vi "BinaryAnalysis.vi"() -> ()   [LabVIEW 2018]
uses:
  <vilib>/Utility/file.llb/Write Delimited Spreadsheet (DBL).vi
panel:
  in  "Save Data?":bool
  in  "Directory to Save Data":path=path "C:/Users/Cletus/Desktop/VMI Scan/100218"
  in  "File Name":path=path "test.txt"
  in  "Step Size":dbl format="%#_13g"
  in  "Initial WL":dbl format="%#_13g"
  in  "length":i32=1000
  in  "index":i32
  in  "Custom Marker Colors":u32[](array[colorbox])=[16714752, 16748562, 16773418]
  in  "Update Marker Colors":bool
  out "Intensity Graph":dbl[][](graph)
  in  "Number of Points/Scan":i32
  out "Waveform Graph":waveform(dbl)(graph)
  out "error out":errorcluster
  in  "Binary File Location (.dat)":path
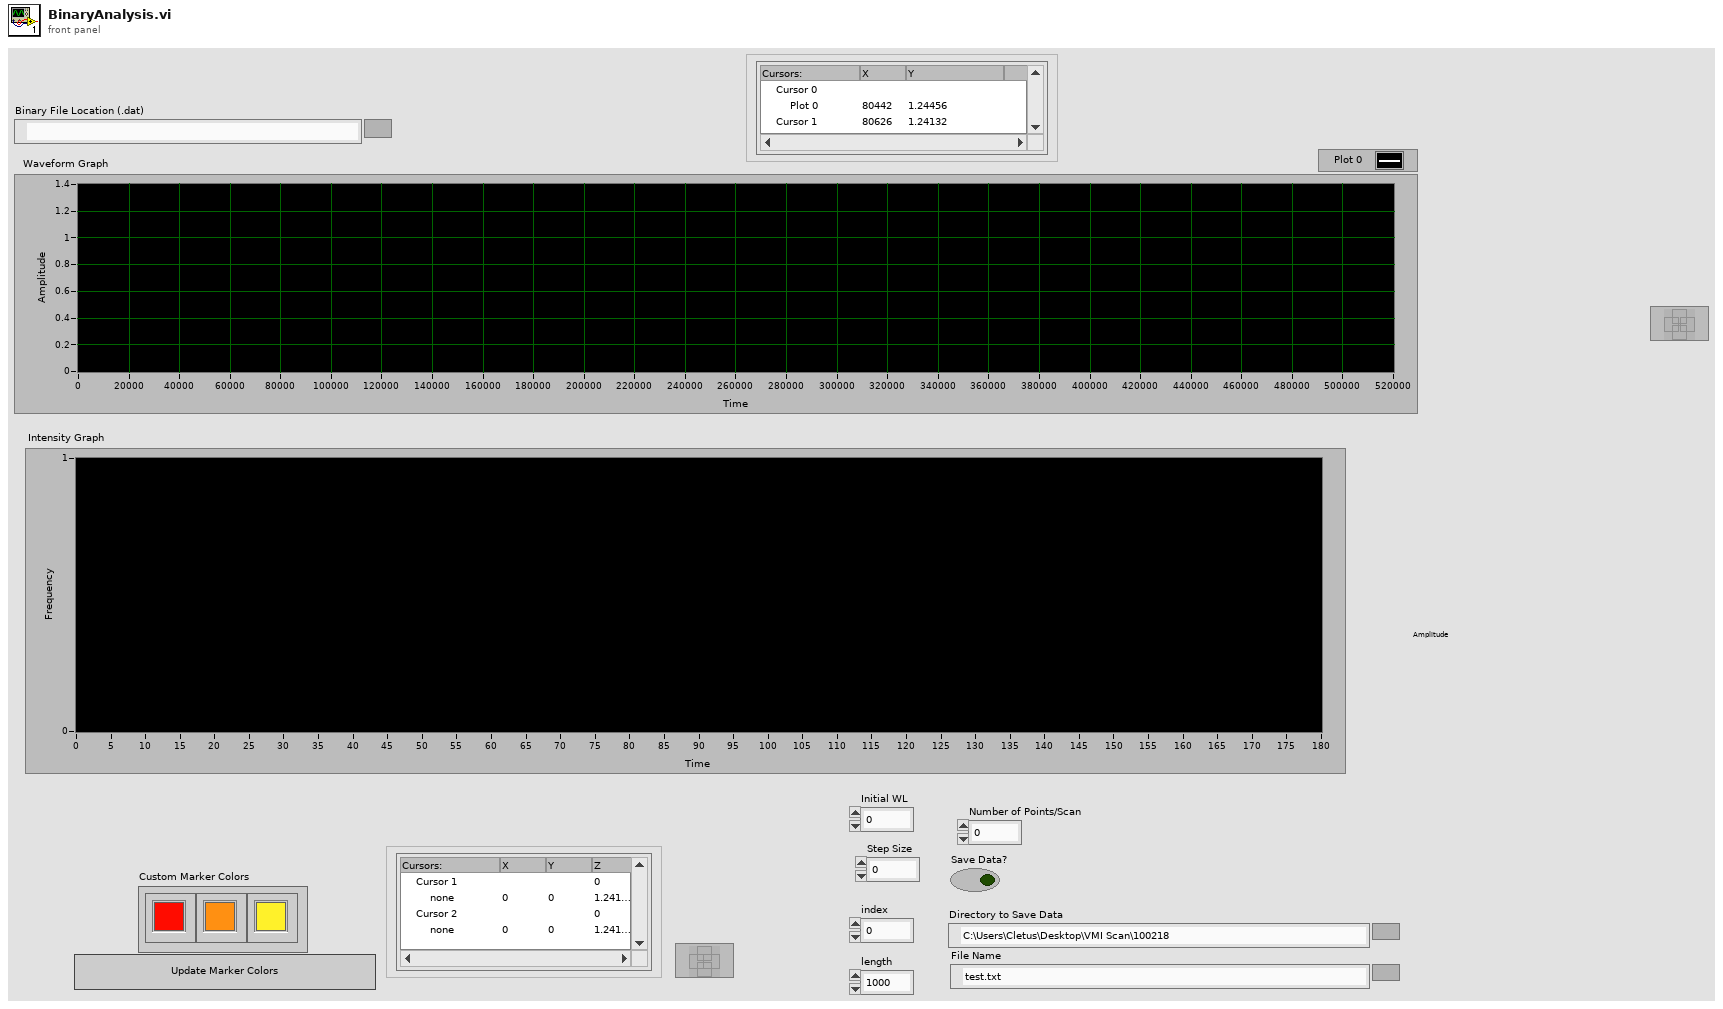
[diagram p1: front panel]
types:
  T1 = enum16{"open", "replace", "create", "open or create", "replace or create", "replace or create with confirmation"}
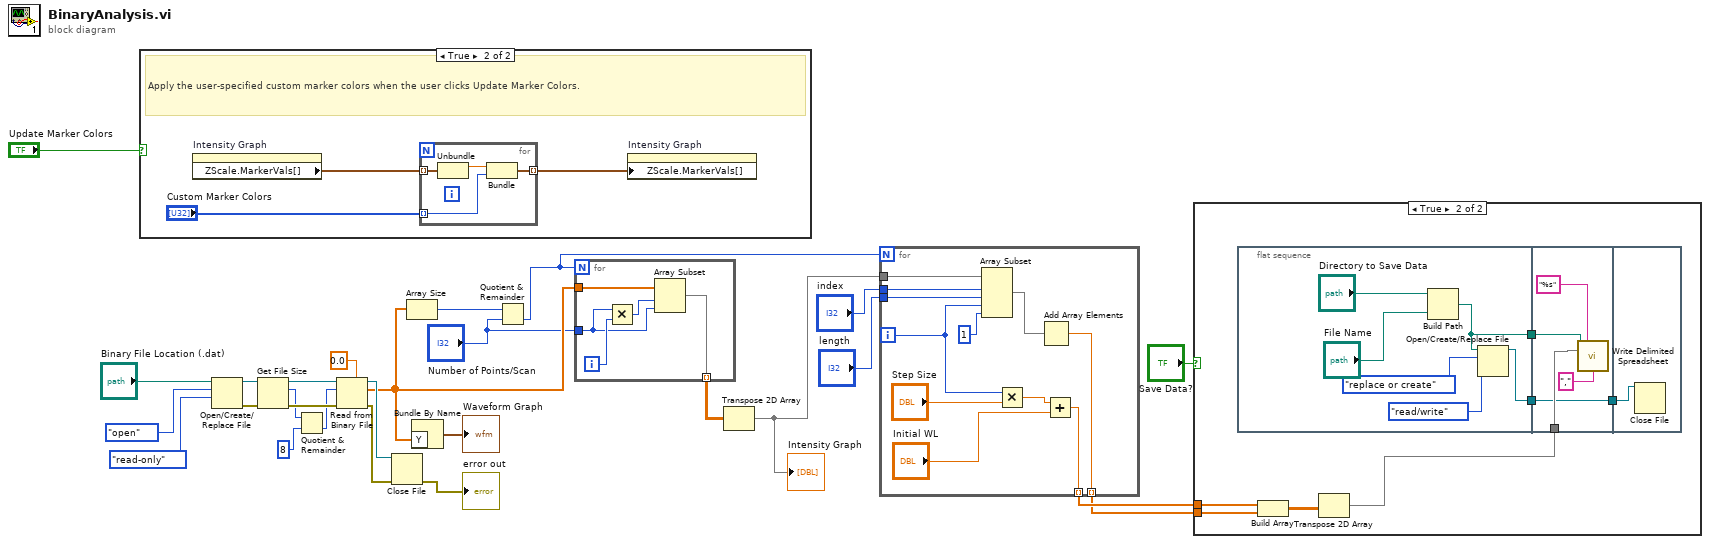
[diagram p0: block diagram]
diagram:
  n1 = case shown="True" "Update Marker Colors" {
    frame False {
      # "Do not manipulate the marker colors if the user has not pressed Update Marker Colors."
    }
    frame True {
      # "Apply the user-specified custom marker colors when the user clicks Update Marker Colors."
      n2 = property on="Intensity Graph" class="IntensityGraph (strict)"() -> ("ZScale.MarkerVals[]"=w30:cluster{dbl, u32}[])  [unwired: 2 in, 2 out]
      n3 = for {
        tunnel: w30 -> [w34] mode=indexing
        tunnel: "Custom Marker Colors" -> [w32] mode=indexing
        tunnel: [w31] -> w28 mode=indexing
        n4 = Unbundle(w34) -> (w33:dbl)  [unwired: 1 out]
        n5 = Bundle(w33, "Color Box"=w32) -> (w31:cluster{dbl, "Color Box":u32})  [unwired: 1 in]
      }
      n6 = property on="Intensity Graph" class="IntensityGraph (strict)"("ZScale.MarkerVals[]"=w28) -> ()  [unwired: 2 in, 2 out]
    }
  }
  n7 = Open/Create/Replace File(file path (use dialog)="Binary File Location (.dat)", operation (0:open)=T1."open", access (0:read/write)=enum16{"read/write", "read-only", "write-only"}."read-only") -> (refnum out=w23:refnum<file>, error out=w24:errorcluster)  [unwired: 3 in, 1 out]
  n8 = Get File Size(file=w23, error in=w24) -> (refnum out=w22:refnum<file>, size (in bytes)=w20:i64, 0:w21:errorcluster)
  n9 = Quotient & Remainder(x=w20, y=i64 8) -> (floor(x/y)=w18:i64)  [unwired: 1 out]
  n10 = Read from Binary File(5:0.0, 8:w21, 10:w18, 11:w22) -> (0:w15:errorcluster, 2:w11:dbl[], 3:w16:refnum<file>)  [unwired: 2 in, 1 out]
  n11 = Close File(refnum=w16, error in=w15) -> (error out=→"error out":errorcluster)  [unwired: 1 out]
  n12 = Array Size(array=w11) -> (size(s)=w12:i32)
  n13 = Bundle By Name("Y"=w11) -> (→"Waveform Graph":waveform(dbl))  [unwired: 1 in]
  n14 = Quotient & Remainder(x=w12, y="Number of Points/Scan") -> (floor(x/y)=w5:i32)  [unwired: 1 out]
  n15 = for {
    N: w5 -> [_]
    tunnel: w11 -> [w39]
    tunnel: "Number of Points/Scan" -> [w36]
    tunnel: [w35] -> w9 mode=indexing
    i -> [w38]
    n16 = Multiply(x=w36, y=w38) -> (x*y=w37:i32)
    n17 = Array Subset(array=w39, index=w37, length=w36) -> (w35:dbl[])
  }
  n18 = Transpose 2D Array(2D array=w9) -> (transposed array=w1:dbl[][])
  "Intensity Graph" <- w1
  n19 = for {
    N: w5 -> [_]
    tunnel: "index" -> [w50]
    tunnel: "length" -> [w49]
    tunnel: w1 -> [w48]
    tunnel: [w42] -> w4 mode=indexing
    tunnel: [w41] -> w3 mode=indexing
    i -> [w46]
    n20 = Array Subset(array=w48, index (row)=w50, length (row)=w49, index (col)=w46, length (col)=1 ("length")) -> (w40:dbl[][])
    n21 = Multiply(x=w46, y="Step Size") -> (x*y=w44:dbl)
    n22 = Add Array Elements(numeric array=w40) -> (sum=w41:dbl)
    n23 = Add(x=w44, y="Initial WL") -> (x+y=w42:dbl)
  }
  n24 = case shown="True" "Save Data?" {
    tunnel: w4 -> [_ w54]
    tunnel: w3 -> [_ w53]
    frame False {
    }
    frame True {
      n25 = flat-sequence {
        tunnel: [w61] -> w57
        tunnel: [w59] -> w56
        tunnel: w57 -> [w68]
        tunnel: w51 -> [w66]
        tunnel: [w64] -> w55
        tunnel: w56 -> [w64]
        tunnel: w55 -> [w69]
        frame #0 {
          n26 = Build Path(base path="Directory to Save Data", name or relative path="File Name") -> (appended path=w61:path)
          n27 = Open/Create/Replace File(file path (use dialog)=w61, operation (0:open)=T1."replace or create", access (0:read/write)=enum16{"read/write", "read-only", "write-only"}."read/write") -> (refnum out=w59:refnum<file>)  [unwired: 3 in, 2 out]
        }
        frame #1 {
          n28 = call-poly <vilib>:"Write Delimited Spreadsheet.vi"("file path (dialog if empty)"=w68, "format (%.3f)"="%s", "2D data"=w66, "delimiter (\\t)"="," ("delimiter (\\t)")) -> ()  [unwired: 10 in, 2 out]
        }
        frame #2 {
          n29 = Close File(refnum=w69) -> ()  [unwired: 1 in, 2 out]
        }
      }
      n30 = Build Array(w54, w53) -> (w52:dbl[][])
      n31 = Transpose 2D Array(2D array=w52) -> (transposed array=w51:dbl[][])
    }
  }
